vi "obj_DataLog Databases.vi"(0 "method":T3, 1 "databases config {initialize}":cluster{"mode":T2, "path":path}[](array[cluster]), 7 "database (current)":string, 11 "error in (no error)":errorcluster) -> (4 "database ref":T1, 8 "database names":string[](array[string]), 15 "error out":errorcluster)   [LabVIEW 2012]
doc: "Holds a list of database path and names as well as references to per-database info object instances. This object must be initialized from a context that remains in existence for the duration of its use or else the object instances get collected. Its error messages assume that this context is a module script of the \"Databases Module\"."
uses:
  typedefs/t_DataLog Databases Methods.ctl
  typedefs/t_DataLog Database Info Pane.ctl
  typedefs/t_Datalog Datebase Modes.ctl
  typedefs/t_DataLog Mirror State Methods.ctl
  typedefs/t_DataLog Tag Info List Methods.ctl
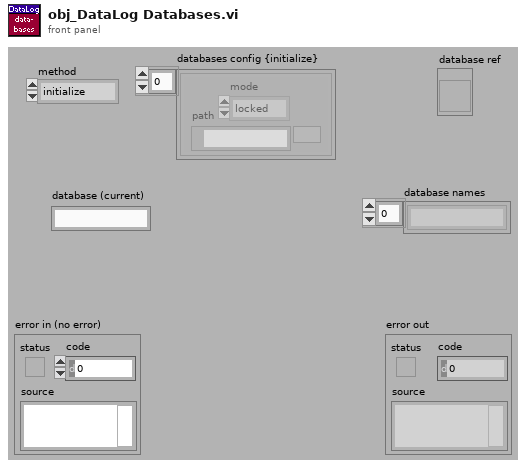
[diagram p1: front panel]
types:
  T1 = typedef "t_DataLog Database Info Pane.ctl" = refnum<vi>
  T2 = typedef "t_Datalog Datebase Modes.ctl" = enum16{"locked", "unlocked", "live", "mirrored"}
  T3 = typedef "t_DataLog Databases Methods.ctl" = enum16{"initialize", "get ref", "get names", "cleanup"}
  T4 = typedef "t_DataLog Mirror State Methods.ctl" = enum16{"add db", "check db", "set", "get", "unset", "clear"}
  T5 = typedef "t_DataLog Tag Info List Methods.ctl" = enum16{"initialize", "create", "create empty", "rename", "delete", "test tag", "get", "get by name", "get default", "get list", "get path", "get subsets", "set subsets", "set config", "set capacity", "#tags", "go live", "set unlocked", "set mirrored"}
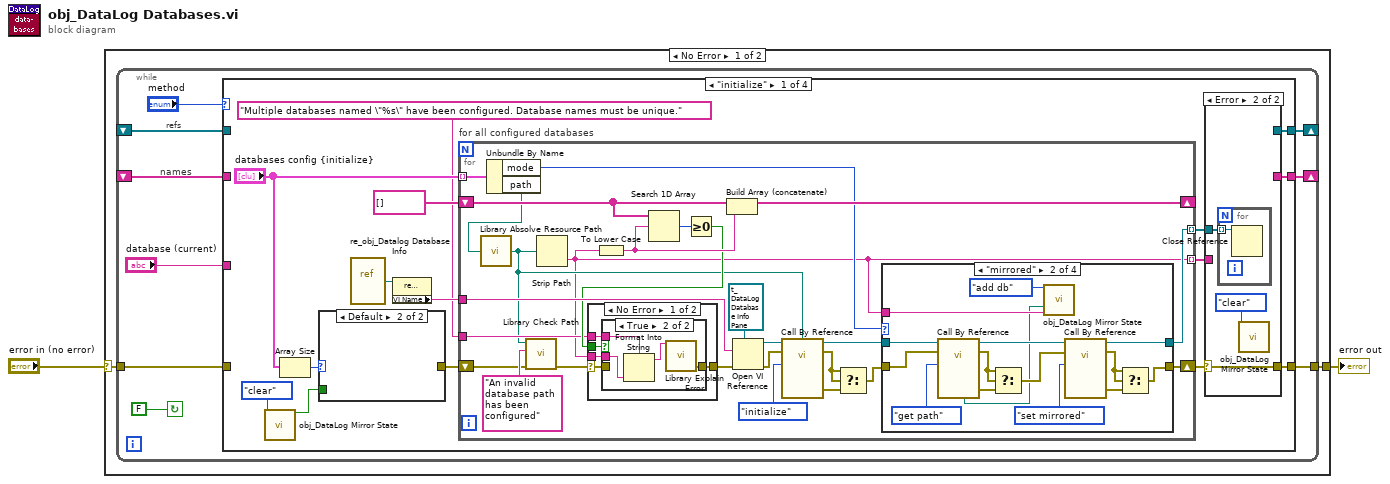
[diagram p0: block diagram]
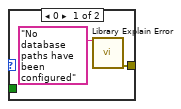
[diagram p3: hidden frame]
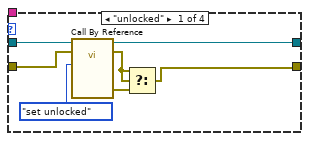
[diagram p4: hidden frame]
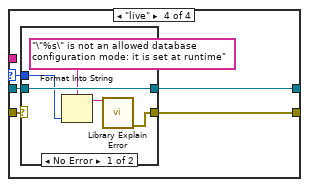
[diagram p6: hidden frame]
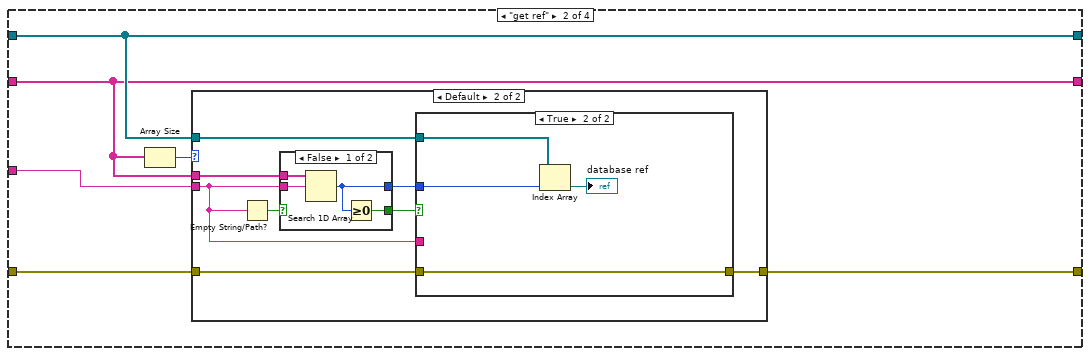
[diagram p10: hidden frame]
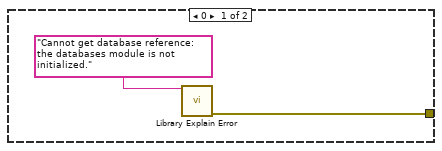
[diagram p11: hidden frame]
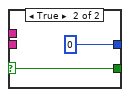
[diagram p12: hidden frame]
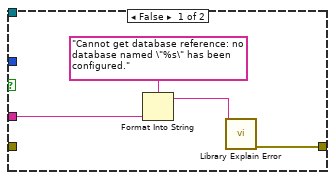
[diagram p13: hidden frame]
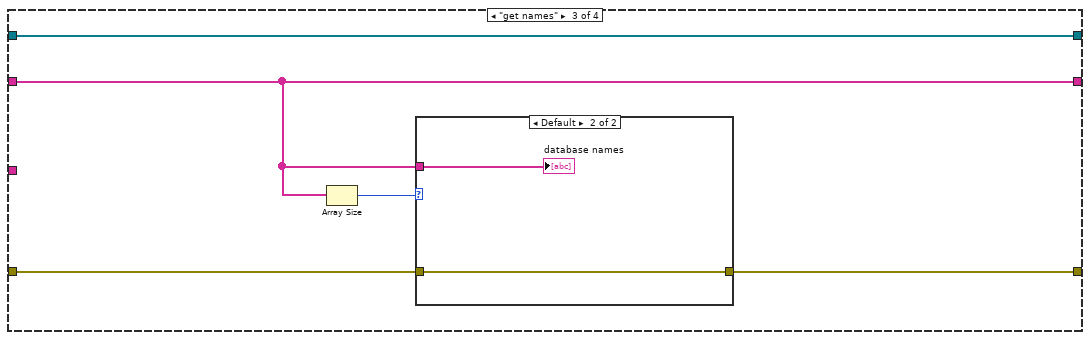
[diagram p14: hidden frame]
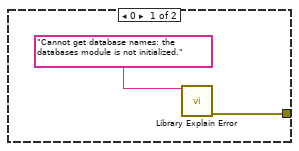
[diagram p15: hidden frame]
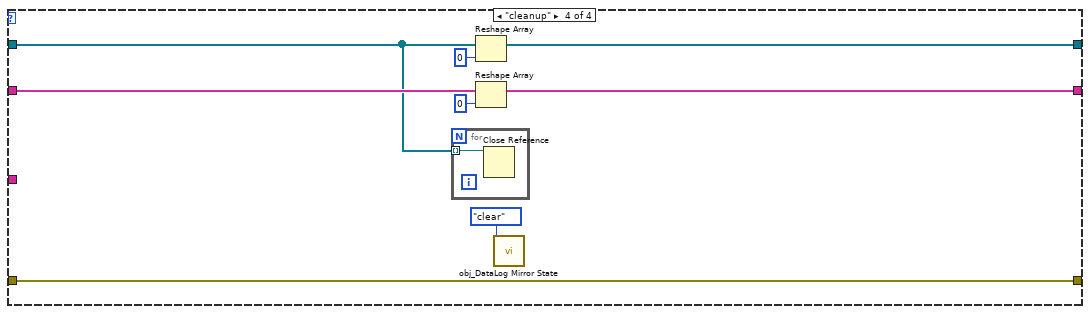
[diagram p16: hidden frame]
diagram:
  n1 = case shown="No Error" "error in (no error)" {
    selector: "error in (no error)" -> [w3 w159]
    tunnel: [w4 w159] -> w1
    frame No Error {
      n2 = while {
        tunnel: [w11] -> w4
        shift-right: [w10] -> _
        shift-left: _ -> [w9]
        shift-right: [w8] -> _
        shift-left: _ -> [w7]
        tunnel: w3 -> [w6]
        stop <- FALSE continue-if-true
        # "refs"
        # "names"
        n3 = case shown="\"initialize\"" "method" {
          tunnel: [w23 w116 w145 w151] -> w11
          tunnel: [w20 w111 w141 w156] -> w10
          tunnel: w9 -> [_ w111 w141 w157]
          tunnel: [w21 w115 w144 w153] -> w8
          tunnel: w7 -> [_ w115 w144 w152]
          tunnel: w6 -> [_ w114 w143 w151]
          tunnel: "database (current)" -> [_ w113 _ _]
          frame "initialize" {
            n4 = call "obj_DataLog Mirror State.vi"("method"=t_DataLog_Mirror_State_Methods."clear") -> ("present?"=w14:bool)  [unwired: 9 in, 5 out]
            n5 = Array Size(array="databases config {initialize}") -> (size(s)=w26:i32)
            n6 = case shown="Default" w26 {
              tunnel: [w37 _] -> w25
              tunnel: w14 -> [_ _]
              frame 0 {
                n7 = call "Library Explain Error.vi"("explanation prefix (none)"="No database paths have been configured") -> ("explained error"=w37:errorcluster)  [unwired: 14 in]
              }
              frame Default {
              }
            }
            n8 = vi-ref "re_obj_Datalog Database Info.vi"() -> ("vi reference"=w16:refnum<vi>)
            n9 = property class="re_obj_Datalog Database Info.vi"(reference=w16) -> ("VI Name"=w28:string)  [unwired: 1 in, 2 out]
            n10 = for "for all configured databases" {
              tunnel: "databases config {initialize}" -> [w45] mode=indexing
              shift-right: [w46] -> w24
              shift-left: w25 -> [w61]
              tunnel: [w38] -> w19 mode=indexing
              tunnel: w28 -> [w62]
              tunnel: [w47] -> w22 mode=indexing
              shift-right: [w60] -> _
              shift-left: string[] [] -> [w59]
              tunnel: "Multiple databases named \"%s\" have been configured. Database names must be unique." ("format string") -> [w53]
              n11 = Unbundle By Name(w45) -> ("mode"=w43:T2, "path"=w44:path)
              n12 = call "Library Absolve Resource Path.vi"("path in"=w44) -> ("absolved path"=w50:path)  [unwired: 14 in]
              n13 = call "Library Check Path.vi"("error in (no error)"=w61, "further explanation (none)"="An invalid database path has been configured", "path"=w50) -> ("error out"=w56:errorcluster)  [unwired: 3 in, 1 out]
              n14 = Strip Path(path=w50) -> (name=w38:string)  [unwired: 1 out]
              n15 = To Lower Case(string=w38) -> (all lower case string=w58:string)
              n16 = Search 1D Array(1D array=w59, element=w58) -> (index of element=w57:i32)  [unwired: 1 in]
              n17 = Greater Or Equal To 0?(x=w57) -> (x >= 0?=w54:bool)
              n18 = case shown="No Error" w56 {
                selector: w56 -> [w104 w110]
                tunnel: [w103 w110] -> w55
                tunnel: w54 -> [w102 _]
                tunnel: w38 -> [w101 _]
                tunnel: w53 -> [w100 _]
                frame No Error {
                  n19 = case shown="True" w102 {
                    tunnel: w104 -> [w105 _]
                    tunnel: [w105 w109] -> w103
                    tunnel: w101 -> [_ w107]
                    tunnel: w100 -> [_ w106]
                    frame False {
                    }
                    frame True {
                      n20 = Format Into String(format string=w106, w107) -> (resulting string=w108:string)  [unwired: 2 in, 1 out]
                      n21 = call "Library Explain Error.vi"("explanation prefix (none)"=w108) -> ("explained error"=w109:errorcluster)  [unwired: 14 in]
                    }
                  }
                }
                frame Error {
                }
              }
              n22 = Build Array (concatenate)(w59, w58) -> (w60:string[])
              n23 = Open VI Reference(type specifier VI Refnum (for type only)=T1 refnum ("tag info list"), vi path=w62, error in (no error)=w55) -> (vi reference=w40:T1, error out=w51:errorcluster)  [unwired: 3 in]
              n24 = call-by-ref "?"(reference=w40, error in=w51, "method"=t_DataLog_Tag_Info_List_Methods."initialize", "database {initialize}"=w50) -> (reference out=w49:T1, error out=w41:errorcluster, 15:"error out"=w42:errorcluster)  [unwired: 7 in, 6 out]
              n25 = Select(t=w41, s=w41, f=w42) -> (s? t:f=w48:errorcluster)
              n26 = case shown="\"mirrored\"" w43 {
                selector: w43 -> [_ _ _ w88]
                tunnel: w49 -> [w69 w75 w87 w91]
                tunnel: w48 -> [w67 w74 w86 w92]
                tunnel: [w68 w84 w87 w90] -> w47
                tunnel: [w66 w83 w86 w89] -> w46
                tunnel: w38 -> [_ w79 _ _]
                frame "unlocked" {
                  n27 = call-by-ref "?"(reference=w69, error in=w67, "method"=t_DataLog_Tag_Info_List_Methods."set unlocked") -> (reference out=w68:T1, error out=w64:errorcluster, 15:"error out"=w65:errorcluster)  [unwired: 8 in, 6 out]
                  n28 = Select(t=w64, s=w64, f=w65) -> (s? t:f=w66:errorcluster)
                }
                frame "mirrored" {
                  n29 = call-by-ref "?"(reference=w75, error in=w74, "method"=t_DataLog_Tag_Info_List_Methods."get path") -> (reference out=w72:T1, error out=w78:errorcluster, "path"=w71:path, 15:"error out"=w77:errorcluster)  [unwired: 8 in, 5 out]
                  n30 = Select(t=w78, s=w78, f=w77) -> (s? t:f=w73:errorcluster)
                  n31 = call "obj_DataLog Mirror State.vi"("method"=t_DataLog_Mirror_State_Methods."add db", "db path in"=w71, "local db"=w79) -> ()  [unwired: 7 in, 6 out]
                  n32 = call-by-ref "?"(reference=w72, error in=w73, "method"=t_DataLog_Tag_Info_List_Methods."set mirrored") -> (reference out=w84:T1, error out=w81:errorcluster, 15:"error out"=w82:errorcluster)  [unwired: 8 in, 6 out]
                  n33 = Select(t=w81, s=w81, f=w82) -> (s? t:f=w83:errorcluster)
                }
                frame "locked" {
                }
                frame "live" {
                  n34 = case shown="No Error" w92 {
                    selector: w92 -> [_ w98]
                    tunnel: w91 -> [w97 w99]
                    tunnel: [w97 w99] -> w90
                    tunnel: [w96 w98] -> w89
                    tunnel: w88 -> [w95 _]
                    frame No Error {
                      n35 = Format Into String(format string="\"%s\" is not an allowed database configuration mode: it is set at runtime", w95) -> (resulting string=w94:string)  [unwired: 2 in, 1 out]
                      n36 = call "Library Explain Error.vi"("explanation prefix (none)"=w94) -> ("explained error"=w96:errorcluster)  [unwired: 14 in]
                    }
                    frame Error {
                    }
                  }
                }
              }
            }
            n37 = case shown="Error" w24 {
              selector: w24 -> [w29 w34]
              tunnel: [w29 w34] -> w23
              tunnel: w22 -> [w31 w33]
              tunnel: [w31 _] -> w21
              tunnel: [w30 _] -> w20
              tunnel: w19 -> [w30 _]
              frame No Error {
              }
              frame Error {
                n38 = for {
                  tunnel: w33 -> [w35] mode=indexing
                  n39 = Close Reference(reference=w35) -> ()  [unwired: 1 in, 1 out]
                }
                n40 = call "obj_DataLog Mirror State.vi"("method"=t_DataLog_Mirror_State_Methods."clear") -> ()  [unwired: 9 in, 6 out]
              }
            }
          }
          frame "get ref" {
            n41 = Array Size(array=w111) -> (size(s)=w112:i32)
            n42 = case shown="Default" w112 {
              tunnel: w111 -> [_ w126]
              tunnel: [w117 w124] -> w116
              tunnel: w115 -> [_ w122]
              tunnel: w114 -> [_ w121]
              tunnel: w113 -> [_ w119]
              frame 0 {
                n43 = call "Library Explain Error.vi"("explanation prefix (none)"="Cannot get database reference: the databases module is not initialized." ("format string")) -> ("explained error"=w117:errorcluster)  [unwired: 14 in]
              }
              frame Default {
                n44 = Empty String/Path?(string/path=w119) -> (empty?=w120:bool)
                n45 = case shown="False" w120 {
                  selector: w120 -> [_ w132]
                  tunnel: w126 -> [w130 _]
                  tunnel: [w129 w132] -> w125
                  tunnel: [w128 0] -> w123
                  tunnel: w119 -> [w127 _]
                  frame False {
                    n46 = Search 1D Array(1D array=w130, element=w127) -> (index of element=w128:i32)  [unwired: 1 in]
                    n47 = Greater Or Equal To 0?(x=w128) -> (x >= 0?=w129:bool)
                  }
                  frame True {
                  }
                }
                n48 = case shown="True" w125 {
                  tunnel: [w136 w137] -> w124
                  tunnel: w123 -> [_ w140]
                  tunnel: w122 -> [_ w139]
                  tunnel: w121 -> [_ w137]
                  tunnel: w119 -> [w135 _]
                  frame False {
                    n49 = Format Into String(format string="Cannot get database reference: no database named \"%s\" has been configured.", w135) -> (resulting string=w133:string)  [unwired: 2 in, 1 out]
                    n50 = call "Library Explain Error.vi"("explanation prefix (none)"=w133) -> ("explained error"=w136:errorcluster)  [unwired: 14 in]
                  }
                  frame True {
                    n51 = Index Array(array=w139, index=w140) -> (element=→"database ref":T1)
                  }
                }
              }
            }
          }
          frame "get names" {
            n52 = Array Size(array=w141) -> (size(s)=w142:i32)
            n53 = case shown="Default" w142 {
              tunnel: [w147 w149] -> w145
              tunnel: w143 -> [_ w149]
              tunnel: w141 -> [_ w148]
              frame 0 {
                n54 = call "Library Explain Error.vi"("explanation prefix (none)"="Cannot get database names: the databases module is not initialized." ("format string")) -> ("explained error"=w147:errorcluster)  [unwired: 14 in]
              }
              frame Default {
                "database names" <- w148
              }
            }
          }
          frame "cleanup" {
            n55 = for {
              tunnel: w152 -> [w158] mode=indexing
              n56 = Close Reference(reference=w158) -> ()  [unwired: 1 in, 1 out]
            }
            n57 = Reshape Array(w152, 0 ("dimension size")) -> (w153:T1[])
            n58 = Reshape Array(w157, 0 ("dimension size")) -> (w156:string[])
            n59 = call "obj_DataLog Mirror State.vi"("method"=t_DataLog_Mirror_State_Methods."clear") -> ()  [unwired: 9 in, 6 out]
          }
        }
      }
    }
    frame Error {
    }
  }
  "error out" <- w1
